vi "Read Tcp Message.vi"(8 "error in (no error)":errorcluster, 9 "bytes to read":i32=5000, 10 "Request Message":u8[](array[numeric]), 11 "Siemens Ctr":T1) -> (0 "error out":errorcluster, 1 "bytes written":i32, 2 "Recieve Message":u8[](array[numeric]), 3 "S7 Connection out":T1)   [LabVIEW 2014, in "Simatic S7.lvlib"]
uses:
  Simatic S7.lvlib
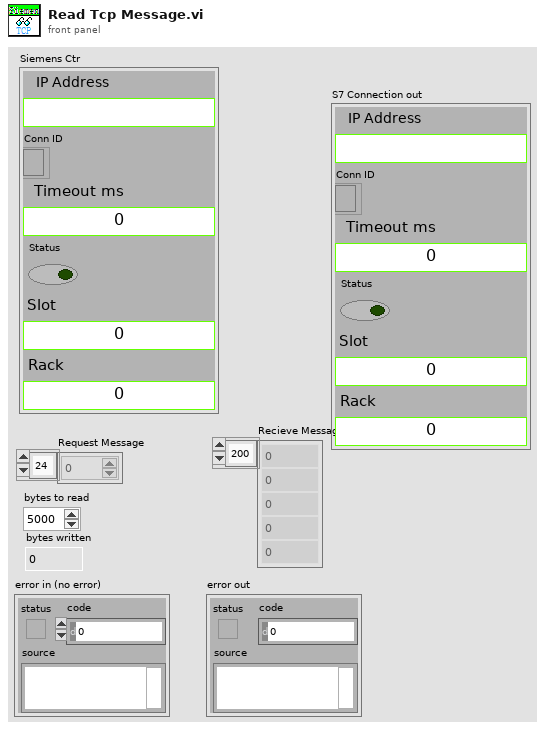
[diagram p1: front panel]
types:
  T1 = typedef "Simatic S7.lvlib/Siemens Ref.ctl" = cluster{"IP Address ":string, "Conn ID":refnum<k5>, "Timeout ms":i32, "Status":bool, "Slot":u16, "Rack":u16}
  T2 = enum16{"Standard", "Buffered", "CRLF", "Immediate"}
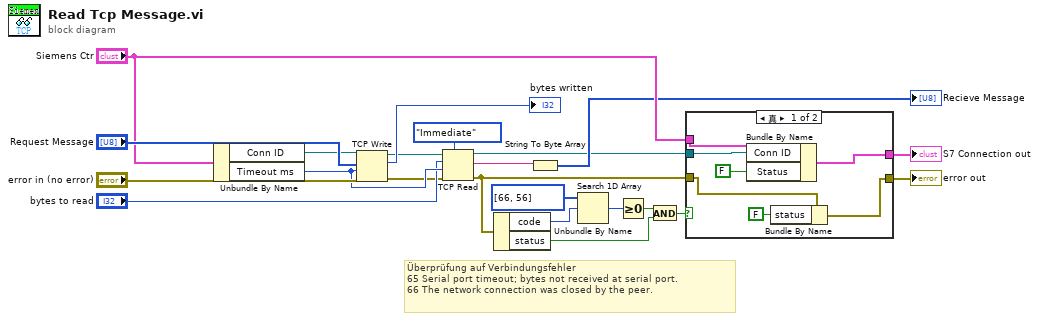
[diagram p0: block diagram]
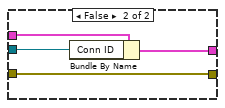
[diagram p2: hidden frame]
diagram:
  # "Überprüfung auf Verbindungsfehler\n65 Serial port timeout; bytes not received at serial port. \n66 The network connection was closed by the peer."
  n1 = Unbundle By Name("Siemens Ctr") -> ("Conn ID"=w9:refnum<k5>, "Timeout ms"=w16:i32)
  n2 = TCP Write(connection ID=w9, data in="Request Message", error in (no error)="error in (no error)", 9:w16) -> (connection ID out=w6:refnum<k5>, bytes written=→"bytes written":i32, error out=w5:errorcluster)
  n3 = TCP Read(connection ID=w6, bytes to read="bytes to read", error in (no error)=w5, 7:T2."Immediate" ("mode (standard)"), 9:w16) -> (connection ID out=w14:refnum<k5>, data out=w17:string, error out=w13:errorcluster)
  n4 = Unbundle By Name(w13) -> ("code"=w3:i32, "status"=w11:bool)
  n5 = String To Byte Array(string=w17) -> (unsigned byte array=→"Recieve Message":u8[])
  n6 = Search 1D Array(1D array=i32[] [66, 56], element=w3) -> (index of element=w1:i32)  [unwired: 1 in]
  n7 = Greater Or Equal To 0?(x=w1) -> (x >= 0?=w2:bool)
  n8 = And(x=w2, y=w11) -> (x .and. y?=w10:bool)
  n9 = case shown="真" w10 {
    tunnel: "Siemens Ctr" -> [w28 w33]
    tunnel: [w24 w32] -> w18
    tunnel: w14 -> [w27 w31]
    tunnel: w13 -> [w26 w30]
    tunnel: [w23 w30] -> w12
    frame True {
      n10 = Bundle By Name(cluster=w28, "Conn ID"=w27, "Status"=FALSE ("Connected?")) -> (w24:T1)
      n11 = Bundle By Name(cluster=w26, "status"=FALSE) -> (w23:errorcluster)
    }
    frame False {
      n12 = Bundle By Name(cluster=w33, "Conn ID"=w31) -> (w32:T1)
    }
  }
  "S7 Connection out" <- w18
  "error out" <- w12
